vi "题目4.vi"() -> ()   [LabVIEW 2017]
uses:
  <vilib>/measure/NI_MABase.lvlib
panel:
  out "Y最大值":dbl
  out "Y大小":i32
  out "Y":dbl[](array[numeric])
  out "dt":dbl
  out "波形图":waveform(dbl)(graph)
  in  "sampling info":cluster{"Fs":dbl, "#s":dbl}={"Fs"=1000.0, "#s"=1000.0} caption="采样信息" {"Fs" format="%.2p"}
  in  "phase":dbl caption="相位" format="%.2p"
  in  "amplitude":dbl=1.0 caption="幅值" format="%.2p"
  in  "frequency":dbl=10.0 caption="频率" format="%.2p"
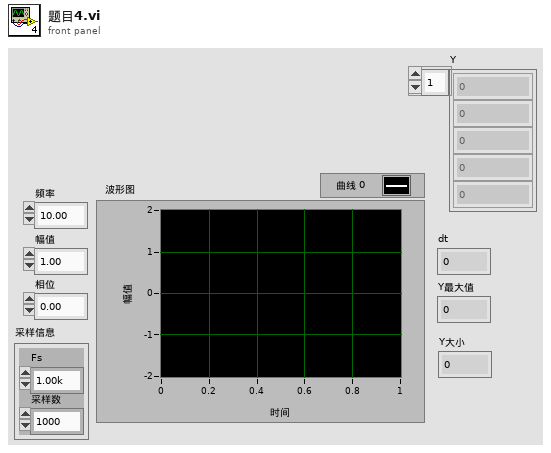
[diagram p1: front panel]
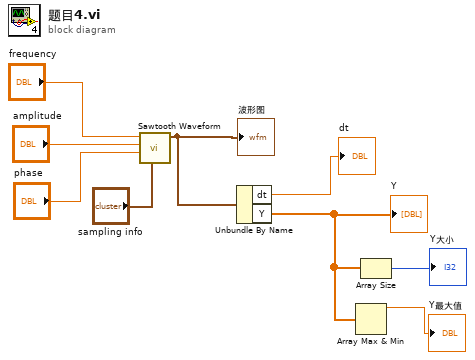
[diagram p0: block diagram]
diagram:
  n1 = call <vilib>:"Sawtooth Waveform.vi"("sampling info"="sampling info", "phase"="phase", "amplitude"="amplitude", "frequency"="frequency") -> ("signal out"=w1:waveform(dbl))  [unwired: 6 in, 1 out]
  "波形图" <- w1
  n2 = Unbundle By Name(w1) -> ("dt"=→"dt":dbl, "Y"=w3:dbl[])
  "Y" <- w3
  n3 = Array Max & Min(array=w3) -> (max value=→"Y最大值":dbl)  [unwired: 3 out]
  n4 = Array Size(array=w3) -> (size(s)=→"Y大小":i32)
